vi "1820 PS Heat duration.vi"(11 "time stamp":timestamp format="%<%I:%M:%S %p>T") -> (3 "PS Heat on (HH:MM:SS)":dbl format="%<%H:%M:%S>t")   [LabVIEW 2016, in "Instrument.Oxford1820.lvclass"]
uses:
  Instrument.Oxford1820.lvclass
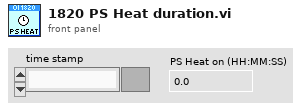
[diagram p1: front panel]
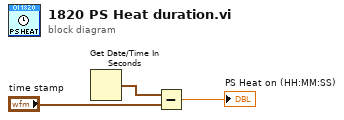
[diagram p0: block diagram]
diagram:
  n1 = Get Date/Time In Seconds() -> (seconds since 1Jan1904=w1:timestamp)
  n2 = Subtract(x=w1, y="time stamp") -> (x-y=→"PS Heat on (HH:MM:SS)":dbl)
